vi "Describe Comparison.vi"(6 "Delta":variant, 8 "error in (no error)":errorcluster, 9 "Actual":variant, 10 "Expected":variant) -> (0 "error out":errorcluster, 2 "Description":string)   [LabVIEW 2020, in "LUnit Test Case V2.lvclass"]
uses:
  LUnit Test Case V2.lvclass
  <vilib>/Utility/Data Type/Get Type Information.vi
  <vilib>/Utility/LVClass/Get LV Class Name.vi
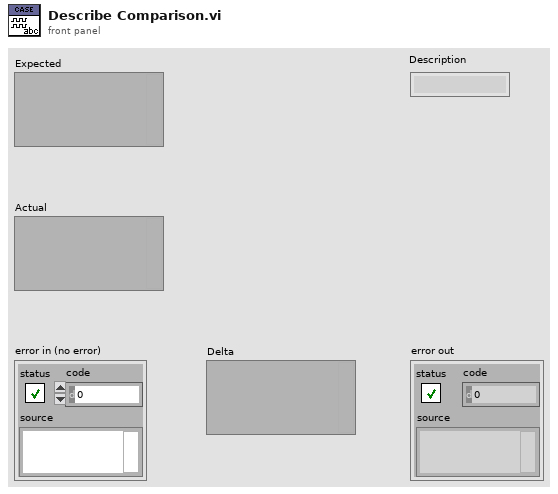
[diagram p1: front panel]
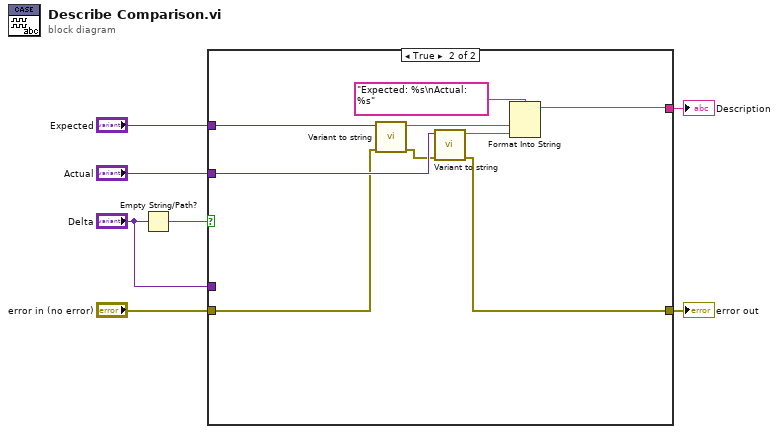
[diagram p0: block diagram]
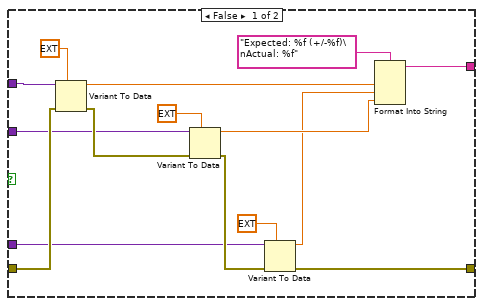
[diagram p2: hidden frame]
diagram:
  n1 = Empty String/Path?(string/path="Delta") -> (empty?=w3:bool)
  n2 = case shown="True" w3 {
    tunnel: "Expected" -> [w14 w28]
    tunnel: "Actual" -> [w9 w27]
    tunnel: "error in (no error)" -> [w13 w25]
    tunnel: [w11 w24] -> w4
    tunnel: "Delta" -> [w10 _]
    tunnel: [w8 w23] -> w1
    frame False {
      n3 = Variant To Data(error in=w13, type=ext 0.0, Variant=w14) -> (data=w17:ext, error out=w19:errorcluster)
      n4 = Variant To Data(error in=w19, type=ext 0.0, Variant=w9) -> (data=w16:ext, error out=w12:errorcluster)
      n5 = Variant To Data(error in=w12, type=ext 0.0, Variant=w10) -> (data=w15:ext, error out=w11:errorcluster)
      n6 = Format Into String(format string="Expected: %f (+/-%f)\nActual: %f", w17, w15, w16) -> (resulting string=w8:string)  [unwired: 2 in, 1 out]
    }
    frame True {
      n7 = call "Variant to string.vi"("error in (no error)"=w25, "Variant"=w28) -> ("error out"=w26:errorcluster, "String"=w31:string)  [unwired: 8 in]
      n8 = call "Variant to string.vi"("error in (no error)"=w26, "Variant"=w27) -> ("error out"=w24:errorcluster, "String"=w29:string)  [unwired: 8 in]
      n9 = Format Into String(format string="Expected: %s\nActual:   %s", w31, w29) -> (resulting string=w23:string)  [unwired: 2 in, 1 out]
    }
  }
  "Description" <- w1
  "error out" <- w4
